vi "MarenGroupGUI.vi"() -> ()   [LabVIEW 2023]
uses:
  <vilib>/Utility/miscctls.llb/LVRowAndColumnTypeDef.ctl
  9ac5065d-0090-4193-bcab-09603eb79785.vi
  d6f1f5d1-b567-48c5-a50c-5634632d964e.vi
  <vilib>/Array/Sort 2D Array - Pop Stack.vi
  <vilib>/Array/Sort 2D Array - Push Stack.vi
  <vilib>/Python/Open Venv Python Session.vi
  <vilib>/Waveform/DWDTOps.llb/DWDT Digital to Analog.vi
panel:
  out "analog waveform":waveform(dbl)
  in  "Tab Control":T1(tab)
  in  "DACs & TTLs":string[][](table)
  out "ADC Analog Voltage":cluster{"Y":dbl[], "Y":dbl[]}[](graph)
  out "ADC Analog Voltage 2":cluster{"Y":dbl[], "Y":dbl[]}[](graph)
  in  "Error Information":string[][](table)
  in  "Input Errors (Disabled)":T2
  out "DAC Error(s)":T2
  out "TTL Error(s)":T2
  out "Simulation LED":bool
  out "Loaded LED":bool
  in  "Protocol File":path
  in  "Start/Stop Button":bool
  in  "Load File Button":bool
  # "Scripted Control System for Bose-Einstein Condesate"
  # "this isnt needed"
  # "Error Information"
  # "Acknowledgements"
  # "2022-2023 Team with Dr. Venkat and Dr. Maren Mossman\nRachelle Childers - EE\nJoaquin de Cabanyes Galindo - ME\nMatthew Gloriani - CS\nAndrew Jockelle - EE\nBlake Lindemeyer - ME\nChristian Picos - EE"
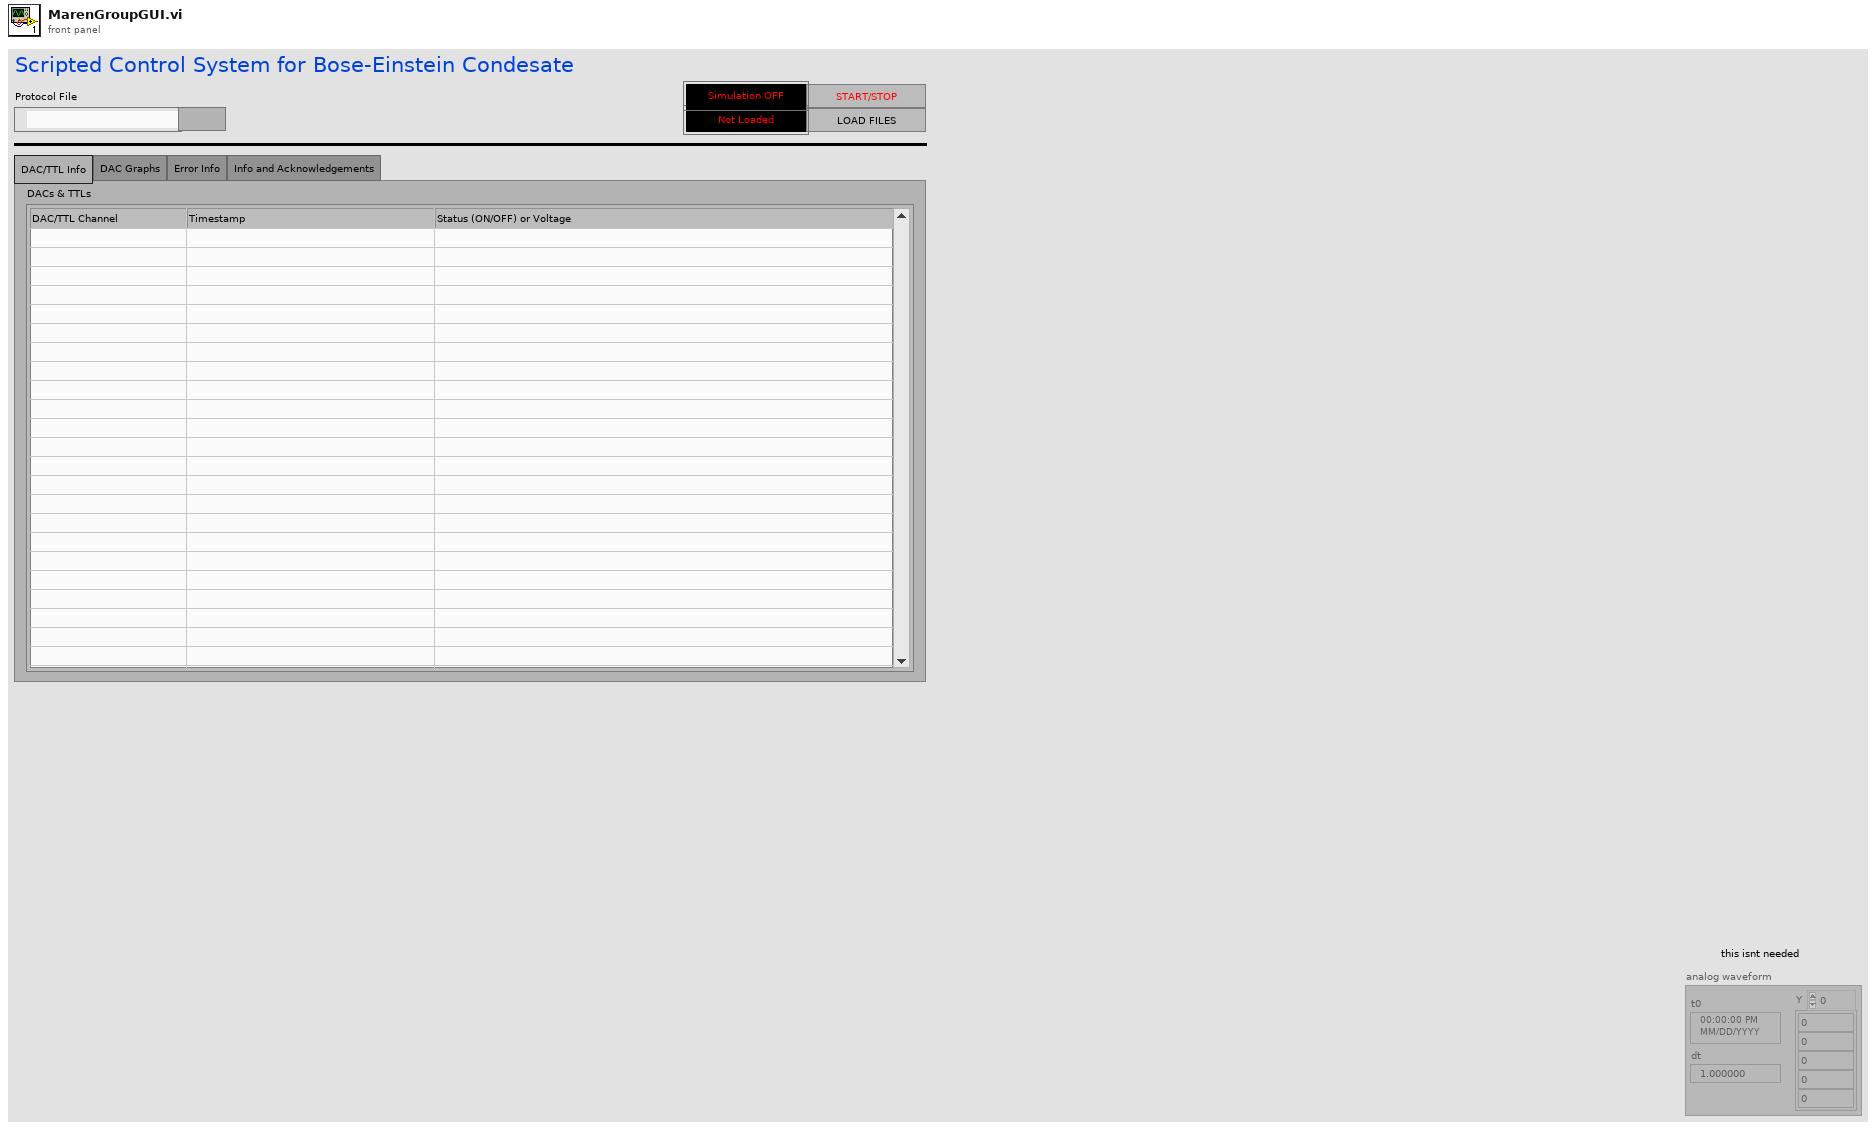
[diagram p1: front panel]
types:
  T1 = enum32{"DAC/TTL Info", "DAC Graphs", "Error Info", "Info and Acknowledgements"}
  T2 = cluster{"status":bool, "number":i32, "description.":string}
  T3 = typedef "LVRowAndColumnTypeDef.ctl" = cluster{"Row":i32, "Column":i32}
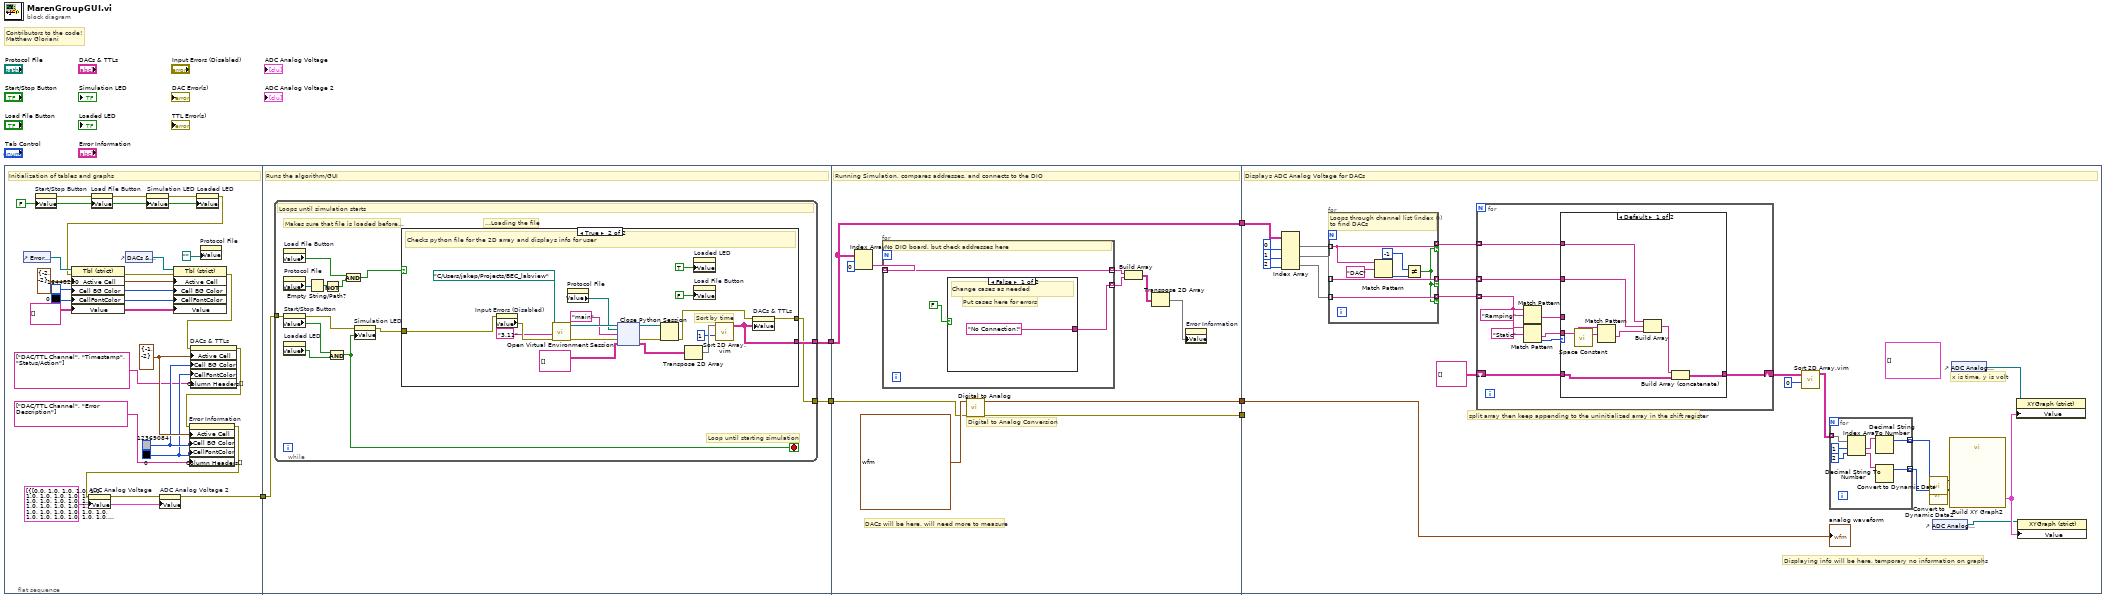
[diagram p0: block diagram]
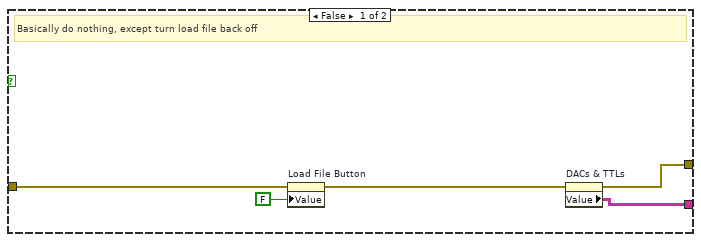
[diagram p2: hidden frame]
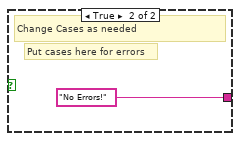
[diagram p3: hidden frame]
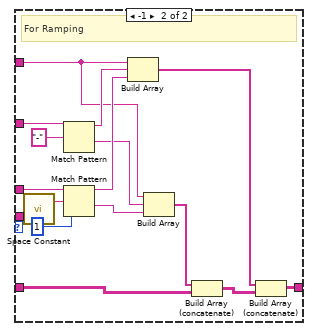
[diagram p4: hidden frame]
diagram:
  # "Contributors to the code!\nMatthew Gloriani"
  n1 = flat-sequence {
    tunnel: [w7] -> w3
    tunnel: [w33] -> w6
    tunnel: w3 -> [w32]
    tunnel: [w31] -> w2
    tunnel: w6 -> [w75]
    tunnel: [w75] -> w5
    tunnel: [w73] -> w4
    tunnel: w2 -> [w72]
    tunnel: [w71] -> w1
    tunnel: w5 -> [w107]
    tunnel: w4 -> [w87]
    tunnel: w1 -> [_]
    frame #0 {
      w9 = cluster{"Y":dbl[], "Y":dbl[]}[] [{"Y"=[0.0, 1.0, 1.0, 1.0, 1.0, 1.0, 1.0, 1.0, 1.0, 1.0, 1.0, 1.0, 1.0, 1.0, 1.0, 1.0, 1.0, 1.0, 1.0, 1.0, 1.0, 1.0, 1.0, 1.0, 1.0, 1.0, 1.0, 1.0, 1.0, 1.0, 1.0, 1.0, 1.0, 1.0, 1.0, 1.0, 1.0, 1.0, 1.0, 1.0, 1.0, 1.0, 1.0, 1.0, 1.0, 1.0, 1.0, 1.0, 1.0, 1.0, 1.0, 1.0, 1.0, 1.0, 1.0, 1.0, 1.0, 1.0, 1.0, 1.0, 1.0, 1.0, 1.0, 1.0, 1.0, 1.0, 1.0, 1.0, 1.0, 1.0], "Y"=[0.0, 3.0, 2.0, 2.0, 2.0, 1.0, 3.0, 1.0, 3.0, 2.0, 2.0, 1.0, 1.0, 2.0, 3.0, 1.0, 1.0, 2.0, 1.0, 2.0, 2.0, 2.0, 2.0, 2.0, 2.0, 1.0, 2.0, 2.0, 2.0, 3.0, 2.0, 1.0, 2.0, 2.0, 2.0, 2.0, 2.0, 2.0, 2.0, 2.0, 1.0, 2.0, 1.0, 3.0, 1.0, 1.0, 2.0, 2.0, 1.0, 3.0, 2.0, 1.0, 2.0, 2.0, 3.0, 2.0, 3.0, 1.0, 1.0, 2.0, 2.0, 2.0, 3.0, 1.0, 2.0, 2.0, 3.0, 1.0, 2.0, 2.0]}] ("ADC Analog Voltage")
      w17 = string[][] [] ("Value")
      w18 = u32 0 ("Active Cell:Cell Font:Color")
      w19 = u32 16448250 ("Active Cell:Cell Background Color")
      w20 = T3 {"Row"=-2, "Column"=-2} ("Active Cell:Active Cell")
      w25 = FALSE ("Start/Stop Button")
      w28 = u32 0 ("Active Cell:Cell Font:Color")
      w29 = u32 12369084 ("Active Cell:Cell Background Color")
      w30 = T3 {"Row"=-1, "Column"=-2} ("Active Cell:Active Cell")
      # "Initialization of tables and graphs"
      n2 = control-ref of="Error Information"() -> (w23:refnum<vi>)
      n3 = property on="Start/Stop Button" class="Bool (strict)"("Value"=w25) -> (error out=w14:errorcluster)  [unwired: 2 in, 1 out]
      n4 = property on="Load File Button" class="Bool (strict)"(error in=w14, "Value"=w25) -> (error out=w13:errorcluster)  [unwired: 1 in, 1 out]
      n5 = control-ref of="DACs & TTLs"() -> (w24:refnum<vi>)
      n6 = property on="Simulation LED" class="Bool (strict)"(error in=w13, "Value"=w25) -> (error out=w12:errorcluster)  [unwired: 1 in, 1 out]
      n7 = property on="Loaded LED" class="Bool (strict)"(error in=w12, "Value"=w25) -> (error out=w11:errorcluster)  [unwired: 1 in, 1 out]
      n8 = property on="Property Node" class="Tbl (strict)"(reference=w23, error in=w11, "Active Cell"=w20, "Cell BG Color"=w19, "CellFontColor"=w18, "Value"=w17) -> (error out=w22:errorcluster)  [unwired: 1 out]
      n9 = property on="Property Node" class="Tbl (strict)"(reference=w24, error in=w22, "Active Cell"=w20, "Cell BG Color"=w19, "CellFontColor"=w18, "Value"=w17) -> (error out=w16:errorcluster)  [unwired: 1 out]
      n10 = property on="DACs & TTLs" class="Tbl (strict)"(error in=w16, "Active Cell"=w30, "Cell BG Color"=w29, "CellFontColor"=w28, "Column Headers[]"=string[] ["DAC/TTL Channel", "Timestamp", "Status/Action"] ("Column Header Strings[]")) -> (error out=w15:errorcluster)  [unwired: 1 in, 1 out]
      n11 = property on="Error Information" class="Tbl (strict)"(error in=w15, "Active Cell"=w30, "Cell BG Color"=w29, "CellFontColor"=w28, "Column Headers[]"=string[] ["DAC/TTL Channel", "Error Description"] ("Column Header Strings[]")) -> (error out=w10:errorcluster)  [unwired: 1 in, 1 out]
      n12 = property on="ADC Analog Voltage" class="XYGraph (strict)"(error in=w10, "Value"=w9) -> (error out=w8:errorcluster)  [unwired: 1 in, 1 out]
      n13 = property on="ADC Analog Voltage 2" class="XYGraph (strict)"(error in=w8, "Value"=w9) -> (error out=w7:errorcluster)  [unwired: 1 in, 1 out]
      n14 = property on="Protocol File" class="Path"("Value"=path "") -> ()  [unwired: 2 in, 2 out]
    }
    frame #1 {
      # "Runs the algorithm/GUI"
      n15 = while {
        tunnel: [w38] -> w33
        tunnel: w32 -> [w36]
        tunnel: [w34] -> w31
        stop <- w39 stop-if-true
        # "...Loading the file"
        # "Makes sure that file is loaded before..."
        # "Loop until starting simulation"
        # "Loops until simulation starts"
        n16 = property on="Load File Button" class="Bool (strict)"() -> ("Value"=w43:bool)  [unwired: 2 in, 2 out]
        n17 = property on="Protocol File" class="Path"() -> ("Value"=w46:path)  [unwired: 2 in, 2 out]
        n18 = property on="Start/Stop Button" class="Bool (strict)"(error in=w36) -> (error out=w35:errorcluster, "Value"=w41:bool)  [unwired: 1 in, 1 out]
        n19 = property on="Loaded LED" class="Bool (strict)"() -> ("Value"=w40:bool)  [unwired: 2 in, 2 out]
        n20 = Empty String/Path?(string/path=w46) -> (empty?=w45:bool)
        n21 = Not(x=w45) -> (.not. x?=w44:bool)
        n22 = And(x=w41, y=w40) -> (x .and. y?=w39:bool)
        n23 = And(x=w43, y=w44) -> (x .and. y?=w42:bool)
        n24 = property on="Simulation LED" class="Bool (strict)"(error in=w35, "Value"=w39) -> (error out=w37:errorcluster)  [unwired: 1 in, 1 out]
        n25 = case shown="True" w42 {
          tunnel: [w50 w56] -> w38
          tunnel: w37 -> [w48 w55]
          tunnel: [w47 w53] -> w34
          frame False {
            # "Basically do nothing, except turn load file back off"
            n26 = property on="Load File Button" class="Bool (strict)"(error in=w48, "Value"=FALSE ("Load File Button")) -> (error out=w49:errorcluster)  [unwired: 1 in, 1 out]
            n27 = property on="DACs & TTLs" class="Tbl (strict)"(error in=w49) -> (error out=w47:errorcluster, "Value"=w50:string[][])  [unwired: 1 in, 1 out]
          }
          frame True {
            # "Sort by time"
            # "Checks python file for the 2D array and displays info for user"
            n28 = property on="Input Errors (Disabled)" class="Clust (strict)"(error in=w55) -> ("Value"=w69:T2)  [unwired: 1 in, 2 out]
            n29 = call-poly <vilib>:"Open Virtual Environment Session.vi"("error in (no error)"=w69, "Python version"="3.11", "Env path"=path "C:/Users/jakep/Projects/BEC_labview") -> ("error out"=w65:errorcluster, "session out"=w68:refnum<k35>)  [unwired: 7 in]
            n30 = property on="Protocol File" class="Path"() -> ("Value"=w62:path)  [unwired: 2 in, 2 out]
            n31 = node(w68, w62, "main" ("function name"), w65, string[][] []) -> (w67:refnum<k35>, w66:errorcluster, w59:string[][])  [unwired: 2 out]
            n32 = Close Python Session(session in=w67, error in=w66) -> (11:w54:errorcluster)
            n33 = Transpose 2D Array(2D array=w59) -> (transposed array=w58:string[][])
            n34 = property on="Loaded LED" class="Bool (strict)"("Value"=TRUE ("Loaded LED")) -> ()  [unwired: 2 in, 2 out]
            n35 = property on="Load File Button" class="Bool (strict)"("Value"=FALSE ("Load File Button")) -> ()  [unwired: 2 in, 2 out]
            n36 = call "Sort 2D Array.vim"("index"=1, "2D array"=w58) -> ("sorted 2D array"=w56:string[][])  [unwired: 8 in, 1 out]
            n37 = property on="DACs & TTLs" class="Tbl (strict)"(error in=w54, "Value"=w56) -> (error out=w53:errorcluster)  [unwired: 1 in, 1 out]
          }
        }
      }
    }
    frame #2 {
      # "Digital to Analog Conversion"
      # "DACs will be here, will need more to measure"
      # "Running Simulation, compares addresses, and connects to the DIO"
      n38 = Index Array(array=w75, index (col)=0 ("disabled index (col)")) -> (element=w80:string[])  [unwired: 1 in]
      n39 = for {
        tunnel: w80 -> [w84] mode=indexing
        tunnel: [w84] -> w79 mode=indexing
        tunnel: [w82] -> w78 mode=indexing
        # "No DIO board, but check addresses here"
        n40 = case shown="False" FALSE {
          tunnel: ["No Connection!" "No Errors!"] -> w82
          frame False {
            # "Put cases here for errors"
            # "Change cases as needed"
          }
          frame True {
            # "Put cases here for errors"
            # "Change Cases as needed"
          }
        }
      }
      n41 = call-poly <vilib>:"Digital to Analog.vi"("error in (no error)"=w72, "digital waveform"=digitalwaveform {"t0"=timestamp(0 s since 1904-01-01), "dt"=0.0, "Y"={"transitions"=[], "data"=[]}, "error"={"status"=FALSE, "code"=37421928, "source"=""}}) -> ("error out"=w71:errorcluster, "analog waveform"=w73:waveform(dbl))  [unwired: 6 in, 2 out]
      n42 = Build Array(w79, w78) -> (w77:string[][])
      n43 = Transpose 2D Array(2D array=w77) -> (transposed array=w76:string[][])
      n44 = property on="Error Information" class="Tbl (strict)"("Value"=w76) -> ()  [unwired: 2 in, 2 out]
    }
    frame #3 {
      (unwired) cluster{"Y":dbl[], "Y":dbl[]}[] [] ("Value")
      # "Displaying info will be here, temporary no information on graphs"
      # "split array then keep appending to the uninitialized array in the shift register"
      # "x is time, y is volt"
      # "Displays ADC Analog Voltage for DACs"
      n45 = Index Array(array=w107, index (col) #1=0 ("disabled index (col)"), index (col) #2=1 ("index (col)"), index (col) #3=2 ("index (col)")) -> (element #1=w103:string[], element #2=w102:string[], element #3=w101:string[])  [unwired: 3 in]
      n46 = for {
        tunnel: w103 -> [w150] mode=indexing
        tunnel: w102 -> [w155] mode=indexing
        tunnel: w101 -> [w154] mode=indexing
        tunnel: [w155] -> w99 mode=indexing if=w149
        tunnel: [w154] -> w100 mode=indexing if=w149
        tunnel: [w150] -> w98 mode=indexing if=w149
        # "Loops through channel list (index 0) to find DACs"
        n47 = Match Pattern(string=w150, regular expression="DAC") -> (offset past match=w152:i32)  [unwired: 1 in, 3 out]
        n48 = Not Equal?(x=-1, y=w152) -> (x != y?=w149:bool)
      }
      n49 = for {
        tunnel: w100 -> [w122] mode=indexing
        tunnel: w99 -> [w119] mode=indexing
        tunnel: w98 -> [w117] mode=indexing
        shift-right: [w116] -> w96
        shift-left: string[][] [] -> [w118]
        n50 = Match Pattern(string=w122, regular expression="Ramping") -> (after substring=w120:string)  [unwired: 1 in, 3 out]
        n51 = Match Pattern(string=w122, regular expression="Static") -> (after substring=w123:string, offset past match=w125:i32)  [unwired: 1 in, 2 out]
        n52 = case shown="Default" w125 {
          tunnel: w123 -> [w132 _]
          tunnel: w120 -> [_ w145]
          tunnel: w119 -> [w130 w147]
          tunnel: w118 -> [w127 w137]
          tunnel: w117 -> [w131 w139]
          tunnel: [w126 w136] -> w116
          frame Default {
            n53 = call <vilib>:"Space Constant.vi"() -> ("String"=w133:string)
            n54 = Match Pattern(string=w132, regular expression=w133) -> (after substring=w129:string)  [unwired: 1 in, 3 out]
            n55 = Build Array(w131, w130, w129) -> (w128:string[])
            n56 = Build Array (concatenate)(w128, w127) -> (w126:string[][])
          }
          frame -1 {
            # "For Ramping"
            n57 = call <vilib>:"Space Constant.vi"() -> ("String"=w144:string)
            n58 = Match Pattern(string=w147, regular expression="-") -> (before substring=w146:string, after substring=w140:string)  [unwired: 1 in, 2 out]
            n59 = Match Pattern(string=w145, regular expression=w144, offset (0)=1) -> (before substring=w142:string, after substring=w141:string)  [unwired: 2 out]
            n60 = Build Array(w139, w146, w142) -> (w134:string[])
            n61 = Build Array(w139, w140, w141) -> (w138:string[])
            n62 = Build Array (concatenate)(w138, w137) -> (w135:string[][])
            n63 = Build Array (concatenate)(w134, w135) -> (w136:string[][])
          }
        }
      }
      n64 = call "Sort 2D Array.vim"("index"=0, "2D array"=w96) -> ("sorted 2D array"=w94:string[][])  [unwired: 8 in, 1 out]
      n65 = for {
        tunnel: w94 -> [w115] mode=indexing
        tunnel: [w110] -> w91 mode=indexing
        tunnel: [w109] -> w93 mode=indexing
        n66 = Index Array(array=w115, index #1=1 ("index"), index #2=2 ("index")) -> (element #1=w112:string, element #2=w111:string)
        n67 = Decimal String To Number(string=w111) -> (offset past number=w110:i32)  [unwired: 2 in, 1 out]
        n68 = Decimal String To Number(string=w112) -> (offset past number=w109:i32)  [unwired: 2 in, 1 out]
      }
      n69 = call "Convert to Dynamic Data"("Array"=w93) -> ("Dynamic Data Type"=w92:dynamicdata)  [unwired: 3 in]
      n70 = call "Convert to Dynamic Data2"("Array"=w91) -> ("Dynamic Data Type"=w90:dynamicdata)  [unwired: 3 in]
      n71 = control-ref of="ADC Analog Voltage 2"() -> (w88:refnum<vi>)
      n72 = call "Build XY Graph2"("Y Input"=w90, "X Input"=w92) -> ("XY Graph"=w89:cluster{"X":dbl[], "Y":dbl[]}[])  [unwired: 8 in, 1 out]
      n73 = control-ref of="ADC Analog Voltage"() -> (w108:refnum<vi>)
      n74 = property class="XYGraph (strict)"(reference=w108, "Value"=w89) -> ()  [unwired: 1 in, 2 out]
      n75 = property class="XYGraph (strict)"(reference=w88, "Value"=w89) -> ()  [unwired: 1 in, 2 out]
      "analog waveform" <- w87
    }
  }
